vi "Deploy.vi"(8 "error in (no error)":errorcluster, 11 "PPL in":refnum<class "NI_AB_API_DPPL.lvclass">) -> (0 "error out":errorcluster, 3 "PPL out":refnum<class "NI_AB_API_DPPL.lvclass">)   [LabVIEW 2020, in "NI_AB_API_DPPL.lvclass"]
uses:
  <vilib>/AppBuilder/AB_API/DPPL/NI_AB_API_DPPL.lvclass
  e:/builds/penguin/labview/branches/2020/dev/dist/vi.lib/AppBuilder/AB_API/Build/NI_AB_API_Build.lvclass
  <vilib>/AppBuilder/AB_API/Build/NI_AB_API_Build.lvclass
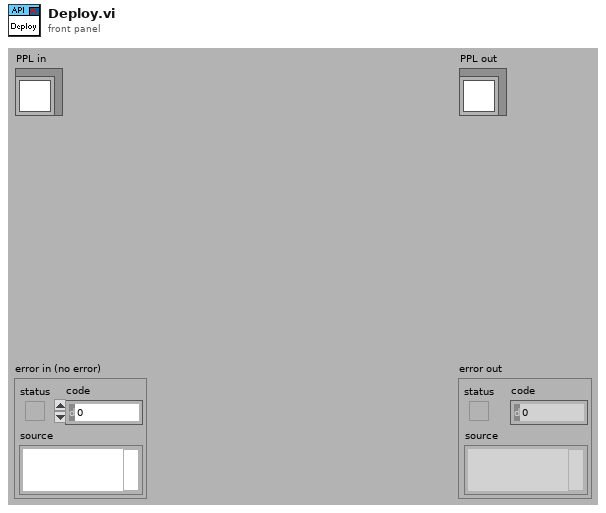
[diagram p1: front panel]
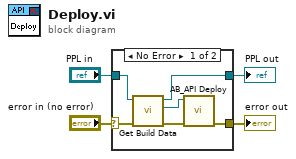
[diagram p0: block diagram]
diagram:
  n1 = case shown="No Error" "error in (no error)" {
    selector: "error in (no error)" -> [w7 w12]
    tunnel: [w10 w12] -> w3
    tunnel: [w8 w11] -> w1
    tunnel: "PPL in" -> [w9 w11]
    frame No Error {
      n2 = call <vilib>:"Get Build Data.vi"("error in (no error)"=w7, "NI_AB_API_Build in"=w9) -> ("error out"=w6:errorcluster, "AB_Build.lvclass"=w5:refnum<class "AB_Build.lvclass">, "NI_AB_API_Build out"=w8:refnum<class "NI_AB_API_DPPL.lvclass">)  [unwired: 7 in]
      n3 = call <vilib>:"AB_API Deploy.vi"("error in (no error)"=w6, "Build in"=w5) -> ("error out"=w10:errorcluster)  [unwired: 8 in, 1 out]
    }
    frame Error {
    }
  }
  "error out" <- w3
  "PPL out" <- w1
